vi "find yellow tote 2d(2).vi"(2 "error in":errorcluster, 3 "Image Src 2":T1) -> (0 "error out 3":errorcluster, 1 "rotation":dbl)   [LabVIEW 2014]
uses:
  <vilib>/vision/Image Controls.llb/IMAQ Image.ctl
  <vilib>/vision/NI_Vision_Development_Module.lvlib
panel:
  out "Image 2":T1(plugin-control)
  out "Image":T1(plugin-control)
  out "Image Out 2":T1(plugin-control)
  out "error out 2":errorcluster
  out "Image Out":T1(plugin-control)
  out "error out":errorcluster
  out "tote":sgl
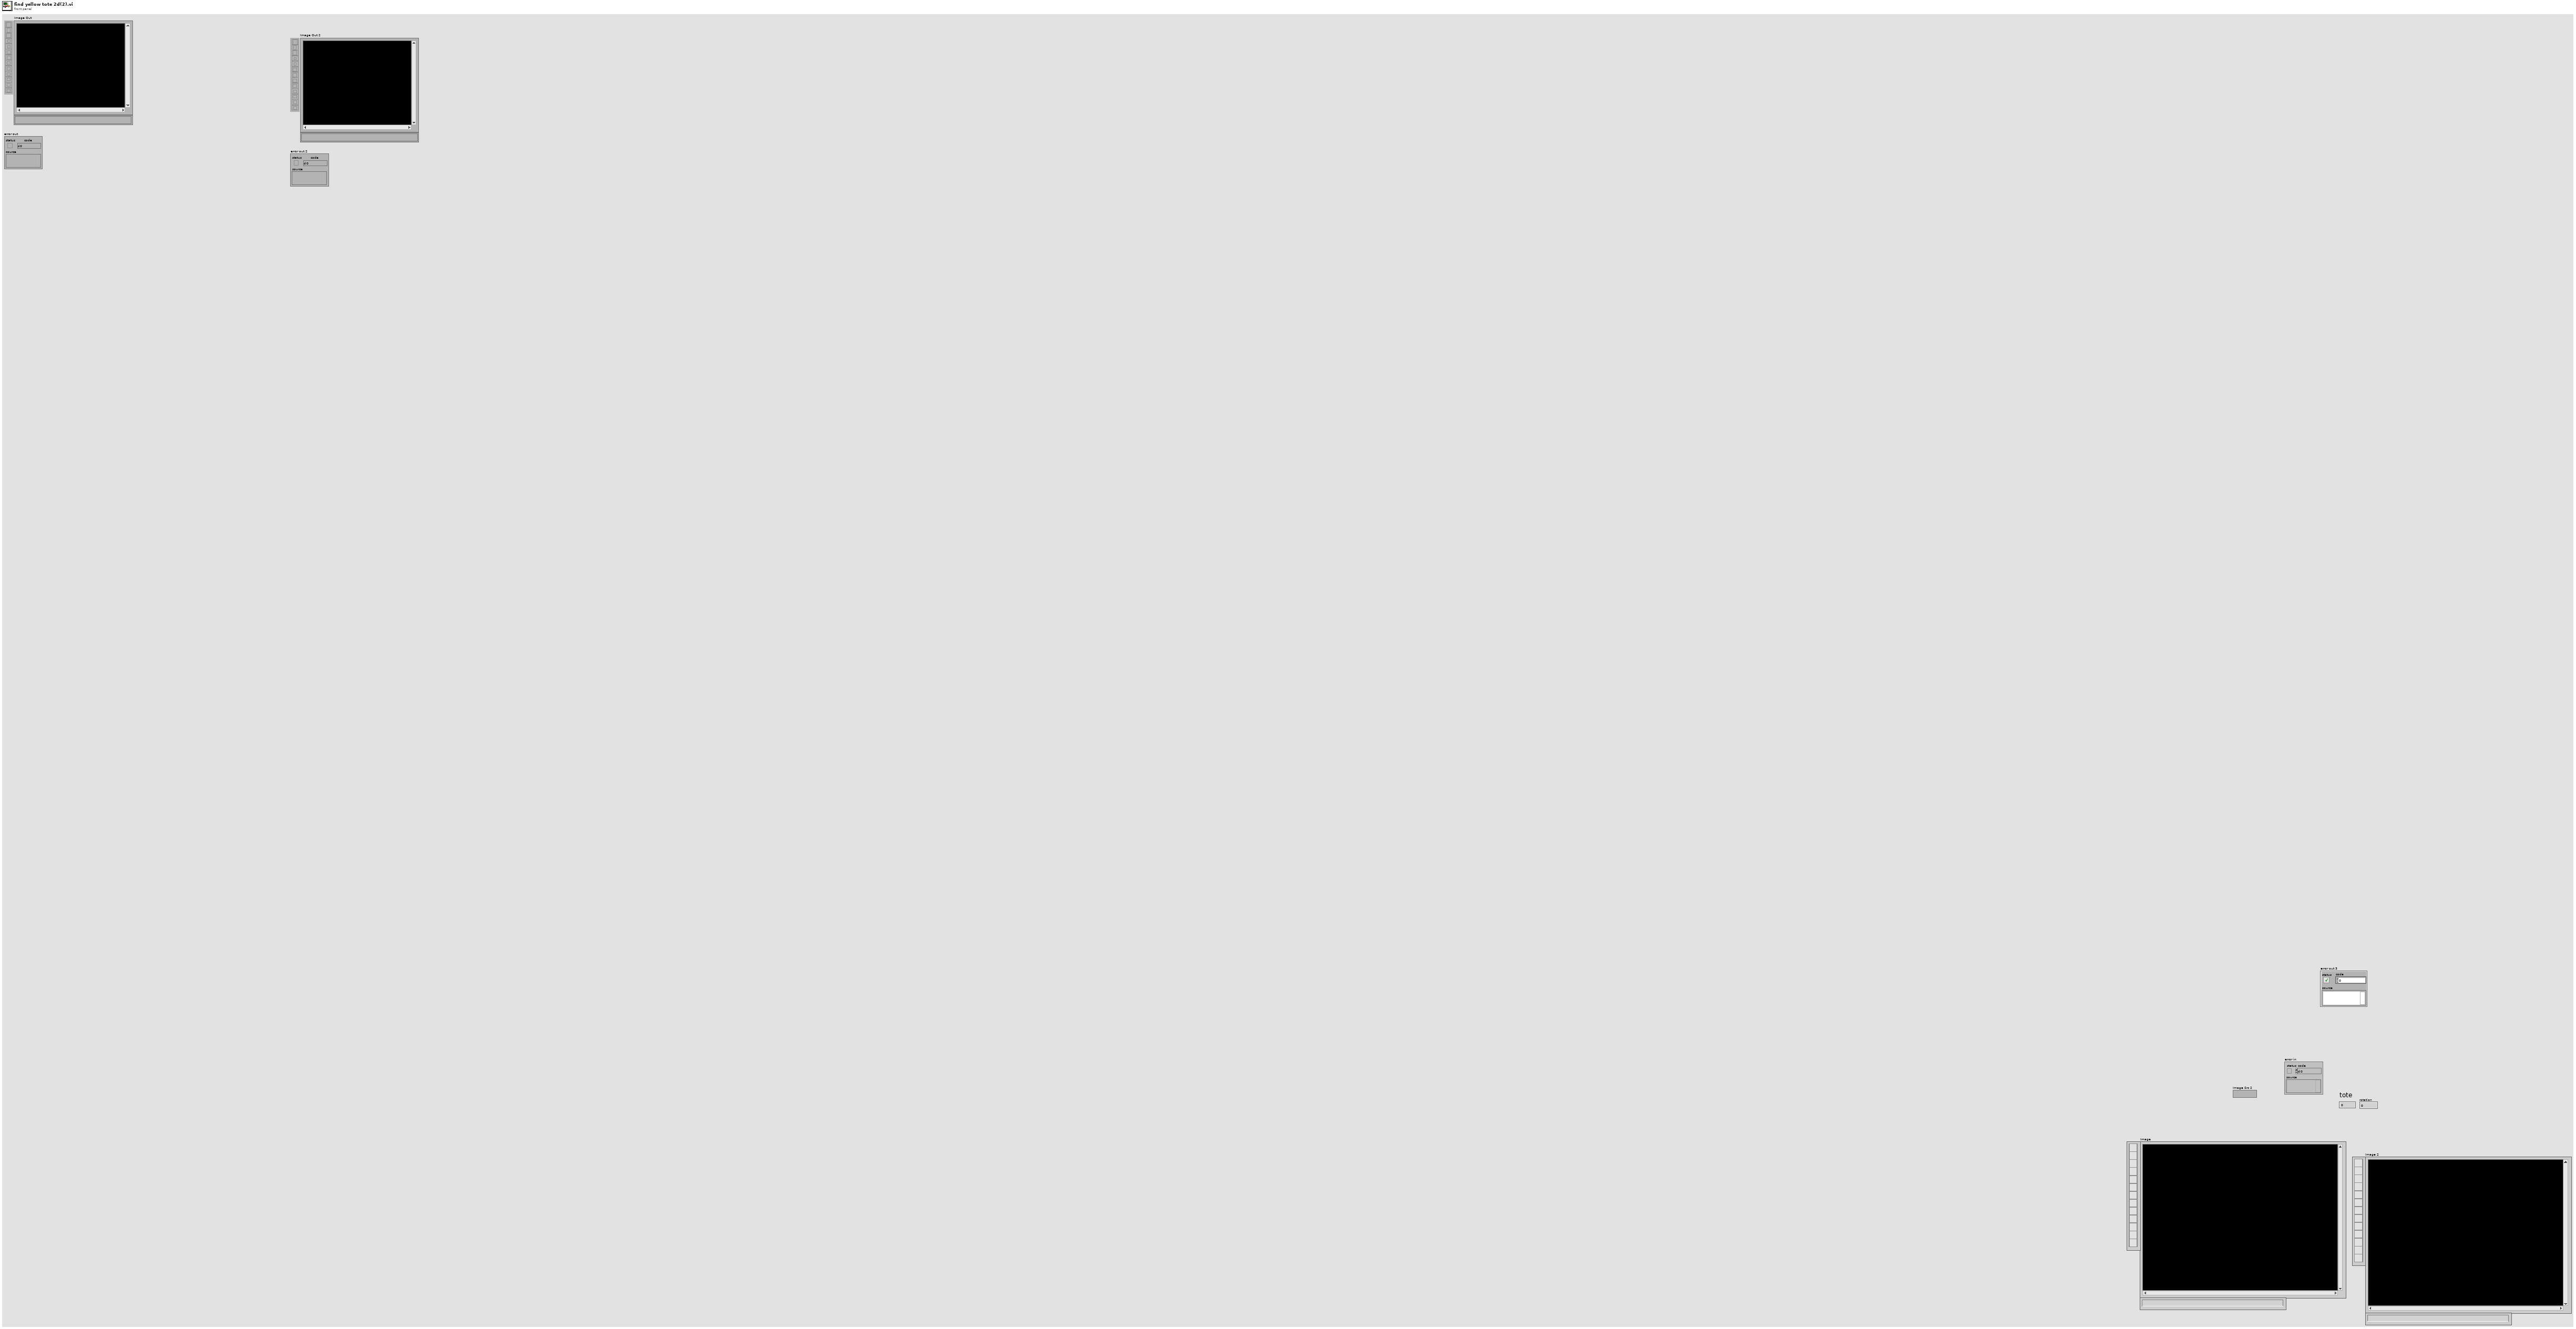
[diagram p1: front panel]
types:
  T1 = typedef "IMAQ Image.ctl" = refnum<image>
  T2 = cluster{"Global Rectangle":i32[], "Contours":cluster{"ID":enum32{"External", "Internal"}, "Type":u32, "Coordinates":i32[]}[]}
  T3 = cluster{"Contrast":i32, "Filter width":i32, "Steepness":i32, "Subsampling Ratio":u32, "Show Search Area":bool, "Show Search Lines":bool, "Show Edges Found":bool, "Show Result":bool}
  T4 = cluster{"ID":enum32{"External", "Internal"}, "Type":u32, "Coordinates":i32[]}[]
  T5 = cluster{"ID":enum32{"External", "Internal"}, "Type":u32, "Coordinates":i32[]}
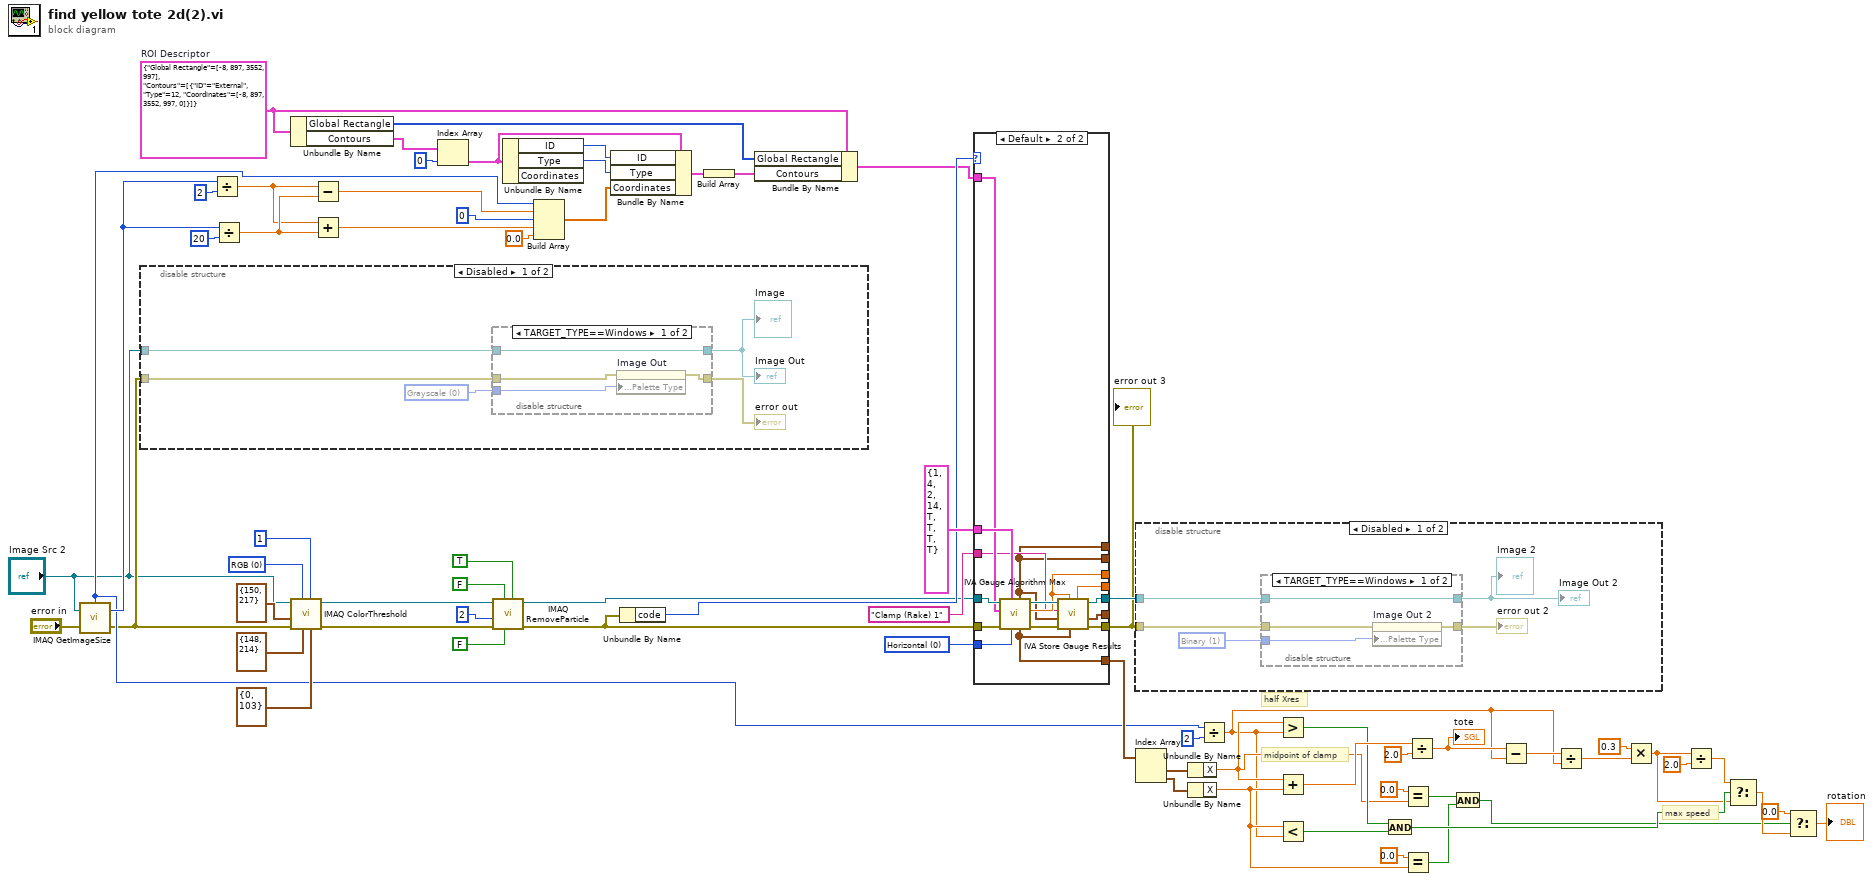
[diagram p0: block diagram]
diagram:
  w44 = T2 {"Global Rectangle"=[-8, 897, 3552, 997], "Contours"=[{"ID"=enum."External", "Type"=12, "Coordinates"=[-8, 897, 3552, 997, 0]}]}  # ROI Descriptor
  w60 = u32 0 items=["Horizontal", "Vertical"] ("Scanning axis")
  w69 = u16 0 items=["RGB", "HSL", "HSV", "HSI"] ("Color Mode")
  # "max speed"
  # "midpoint of clamp"
  # "half Xres"
  n1 = call "IMAQ GetImageSize"("Image"="Image Src 2", "error in (no error)"="error in") -> ("Y Resolution"=w31:i32, "X Resolution"=w29:i32, "error out"=w3:errorcluster)  [unwired: 2 in]
  n2 = disable-structure shown="Disabled" {
    disable-tunnel: "Image Src 2" -> [w73 _]
    disable-tunnel: w3 -> [w72 _]
    frame Disabled {
      w75 = u32 0 items=["Grayscale", "Binary", "Gradient", "Rainbow", "Temperature", "User Defined"] ("Palette")
      n3 = disable-structure "Conditional Disable Structure" shown="TARGET_TYPE==Windows" {
        disable-tunnel: w72 -> [w79 w80]
        disable-tunnel: [w78 w80] -> w71
        disable-tunnel: w73 -> [w77 w81]
        disable-tunnel: [w77 w81] -> w74
        disable-tunnel: w75 -> [w76 _]
        frame condition #0 {
          n4 = property on="Image Out" class="ImageControl"(error in=w79, "Palette:Palette Type"=w76) -> (error out=w78:errorcluster)  [unwired: 1 in, 1 out]
        }
        frame condition #1 (active) {
        }
      }
      "error out" <- w71
      "Image Out" <- w74
      "Image" <- w74
    }
    frame Enabled {
    }
  }
  n5 = Divide(x=w31, y=2) -> (x/y=w54:dbl)
  n6 = Divide(x=w31, y=20) -> (x/y=w55:dbl)
  n7 = Unbundle By Name(w44) -> ("Global Rectangle"=w45:i32[], "Contours"=w53:T4)
  n8 = call "IMAQ ColorThreshold"("Blue or Luma or Val or Inten Range"=cluster{"Lower value":i32, "Upper value":i32} {"Lower value"=0, "Upper value"=103}, "Replace Value"=1, "Green or Sat Range"=cluster{"Lower value":i32, "Upper value":i32} {"Lower value"=148, "Upper value"=214}, "Color Mode"=w69, "error in (no error)"=w3, "Red or Hue Range"=cluster{"Lower value":i32, "Upper value":i32} {"Lower value"=150, "Upper value"=217}, "Image Src"="Image Src 2") -> ("error out"=w12:errorcluster, "Image Dst Out"=w13:T1)  [unwired: 1 in, 2 out]
  n9 = Subtract(x=w54, y=w55) -> (x-y=w41:dbl)
  n10 = Add(x=w54, y=w55) -> (x+y=w43:dbl)
  n11 = Index Array(array=w53, index=0) -> (element=w48:T5)
  n12 = call "IMAQ RemoveParticle"("Connectivity 4/8 (8)"=TRUE, "Low Pass/High Pass (Low)"=FALSE, "Square/Hexa (Square)"=FALSE, "error in (no error)"=w12, "Number of Erosion"=2, "Image Src"=w13) -> ("error out"=w38:errorcluster, "Image Dst Out"=w36:T1)  [unwired: 1 in, 3 out]
  n13 = Unbundle By Name(w48) -> ("ID"=w51:enum32{"External", "Internal"}, "Type"=w50:u32)  [unwired: 1 out]
  n14 = Build Array(w29, w41, 0 ("X1"), w43, 0.0 ("element")) -> (w49:dbl[])
  n15 = Bundle By Name(cluster=w48, "ID"=w51, "Type"=w50, "Coordinates"=w49) -> (w47:T5)
  n16 = Unbundle By Name(w38) -> ("code"=w59:i32)
  n17 = Build Array(w47) -> (w46:T4)
  n18 = Bundle By Name(cluster=w44, "Global Rectangle"=w45, "Contours"=w46) -> (w40:T2)
  n19 = case shown="Default" w59 {
    tunnel: w36 -> [w82 w97]
    tunnel: w38 -> [_ w96]
    tunnel: T3 {"Contrast"=1, "Filter width"=4, "Steepness"=2, "Subsampling Ratio"=14, "Show Search Area"=TRUE, "Show Search Lines"=TRUE, "Show Edges Found"=TRUE, "Show Result"=TRUE} ("Settings") -> [_ w95]
    tunnel: w60 -> [_ w94]
    tunnel: w40 -> [_ w93]
    tunnel: [w82 w91] -> w11
    tunnel: [_ w89] -> w10
    tunnel: [_ w88] -> _
    tunnel: [_ w83] -> _
    tunnel: [_ w87] -> _
    tunnel: [_ w86] -> _
    tunnel: "Clamp (Rake) 1" ("Step Name") -> [_ w85]
    tunnel: [_ w84] -> w37
    tunnel: [_ w83] -> _
    frame -1074396199, -1074396198 {
    }
    frame Default {
      n20 = call <vilib>:"IVA Gauge Algorithm Max.vi"("Scanning axis"=w94, "Settings"=w95, "error in (no error)"=w96, "ROI Descriptor"=w93, "Image"=w97) -> ("error out"=w90:errorcluster, "Distance"=w88:sgl, "Image Out"=w92:T1, "Distance Points"=w84:cluster{"X":sgl, "Y":sgl}[], "Points of Contact"=w83:cluster{"X":sgl, "Y":sgl}[])  [unwired: 1 in, 1 out]
      n21 = call <vilib>:"IVA Store Gauge Results.vi"("Distance Points"=w84, "Distance"=w88, "error in (no error)"=w90, "Points of Contact"=w83, "Step Name"=w85, "Image in"=w92) -> ("error out"=w89:errorcluster, "Points of Contact (calibrated)"=w86:cluster{"X":sgl, "Y":sgl}[], "Image dup"=w91:T1, "Distance (calibrated)"=w87:sgl)  [unwired: 2 out]
    }
  }
  "error out 3" <- w10
  n22 = disable-structure shown="Disabled" {
    disable-tunnel: w11 -> [w100 _]
    disable-tunnel: w10 -> [w99 _]
    frame Disabled {
      w101 = u32 1 items=["Grayscale", "Binary", "Gradient", "Rainbow", "Temperature", "User Defined"] ("Palette")
      n23 = disable-structure "Conditional Disable Structure" shown="TARGET_TYPE==Windows" {
        disable-tunnel: w99 -> [w106 w107]
        disable-tunnel: [w105 w107] -> w102
        disable-tunnel: w100 -> [w104 w108]
        disable-tunnel: [w104 w108] -> w98
        disable-tunnel: w101 -> [w103 _]
        frame condition #0 {
          n24 = property on="Image Out 2" class="ImageControl"(error in=w106, "Palette:Palette Type"=w103) -> (error out=w105:errorcluster)  [unwired: 1 in, 1 out]
        }
        frame condition #1 (active) {
        }
      }
      "error out 2" <- w102
      "Image Out 2" <- w98
      "Image 2" <- w98
    }
    frame Enabled {
    }
  }
  n25 = Index Array(array=w37) -> (element #1=w34:cluster{"X":sgl, "Y":sgl}, element #2=w35:cluster{"X":sgl, "Y":sgl})  [unwired: 2 in]
  n26 = Unbundle By Name(w34) -> ("X"=w14:sgl)
  n27 = Unbundle By Name(w35) -> ("X"=w18:sgl)
  n28 = Divide(x=w29, y=2) -> (x/y=w8:dbl)
  n29 = Greater?(x=w14, y=w8) -> (0:w28:bool)
  n30 = Add(x=w14, y=w18) -> (x+y=w33:sgl)
  n31 = Less?(x=w18, y=w8) -> (x < y?=w27:bool)
  n32 = And(x=w28, y=w27) -> (x .and. y?=w26:bool)
  n33 = Equal?(x=0.0, y=w14) -> (x = y?=w17:bool)
  n34 = Equal?(x=0.0, y=w18) -> (x = y?=w16:bool)
  n35 = Divide(x=w33, y=sgl 2.0) -> (x/y=w25:sgl)
  "tote" <- w25
  n36 = And(x=w17, y=w16) -> (x .and. y?=w15:bool)
  n37 = Subtract(x=w25, y=w8) -> (x-y=w9:dbl)
  n38 = Divide(x=w9, y=w8) -> (x/y=w7:dbl)
  n39 = Multiply(x=0.3, y=w7) -> (x*y=w5:dbl)
  n40 = Divide(x=w5, y=2.0 ("t")) -> (x/y=w4:dbl)
  n41 = Select(t=w4, s=w26, f=w5) -> (s? t:f=w23:dbl)
  n42 = Select(t=0.0, s=w15, f=w23) -> (s? t:f=→"rotation":dbl)
